vi "HL Time to Duty Cycle and Period.vi"(2 "Low Time":dbl, 3 "High Time":dbl) -> (0 "Period":dbl, 1 "Duty Cycle (%)":dbl)   [LabVIEW 2016]
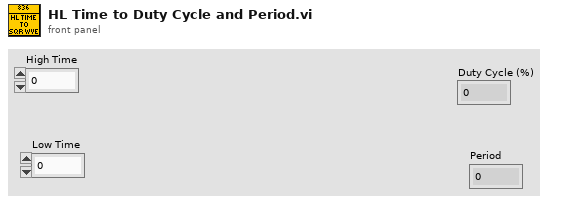
[diagram p1: front panel]
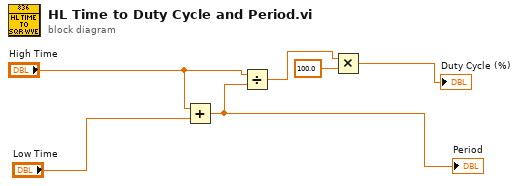
[diagram p0: block diagram]
diagram:
  n1 = Add(x="High Time", y="Low Time") -> (x+y=w3:dbl)
  "Period" <- w3
  n2 = Divide(x="High Time", y=w3) -> (x/y=w4:dbl)
  n3 = Multiply(x=w4, y=100.0) -> (x*y=→"Duty Cycle (%)":dbl)
